vi "Calculate Output Sampling.vi"(10 "sampling info":cluster{"Fs":dbl, "#s":dbl}={"Fs"=204800.0, "#s"=20480.0}, 11 "Cfg_REF":T2 {"Roll-Off" min=1 max=4; "TC" min=1e-06 max=100.0 format="%#_3p"; "Phase" format="%#_3p"; "Frequency" min=1e-06 max=102400.0 format="%#_6p"; "Channel" min=1}) -> (2 "Filter Parameters":T1, 3 "Cfg_REF out":T2 {"Roll-Off" min=1 max=4; "TC" min=1e-06 max=100.0 format="%#_3p"; "Phase" format="%#_3p"; "Frequency" min=1e-06 max=102400.0 format="%#_6p"; "Channel" min=1})   [LabVIEW 2019, in "Instrument.Lockin.lvlib" / "Instrument.Lockin.lvclass"]
uses:
  Instrument.Lockin.lvclass
  Instrument.DAQ/Typedefs/REF.Channel--Cluster--Array.ctl
  Instrument.DAQ/Typedefs/REF.Channel--Cluster.ctl
  DSP/DSP.lvclass
  Instrument.DAQ/Instrument.DAQ.lvclass
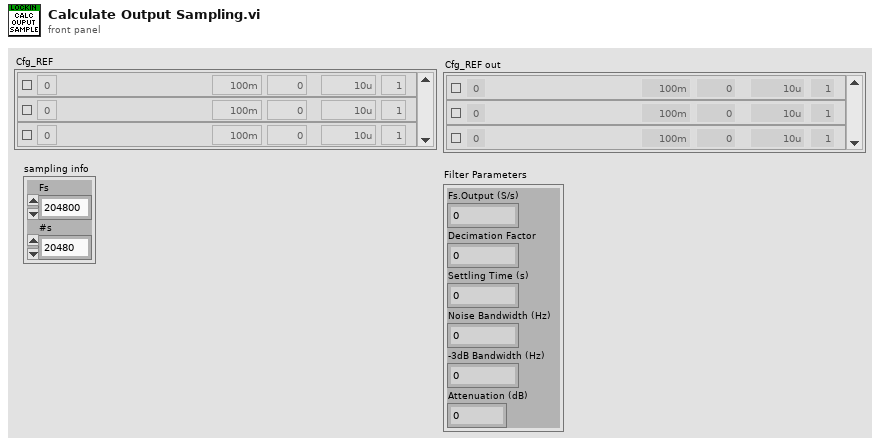
[diagram p1: front panel]
types:
  T1 = cluster{"Fs.Output (S/s)":dbl, "Decimation Factor":i32, "Settling Time (s)":dbl, "Noise Bandwidth (Hz)":dbl, "-3dB Bandwidth (Hz)":dbl, "Attenuation (dB)":dbl}
  T2 = typedef "Instrument.Lockin.lvlib/Instrument.DAQ.lvclass/REF.Channel--Cluster--Array.ctl" = T3[]
  T3 = typedef "Instrument.Lockin.lvlib/Instrument.DAQ.lvclass/REF.Channel--Cluster.ctl" = cluster{"Enable?":bool, "Channel":i32, "Frequency":dbl, "Phase":dbl, "TC":dbl, "Roll-Off":i32}
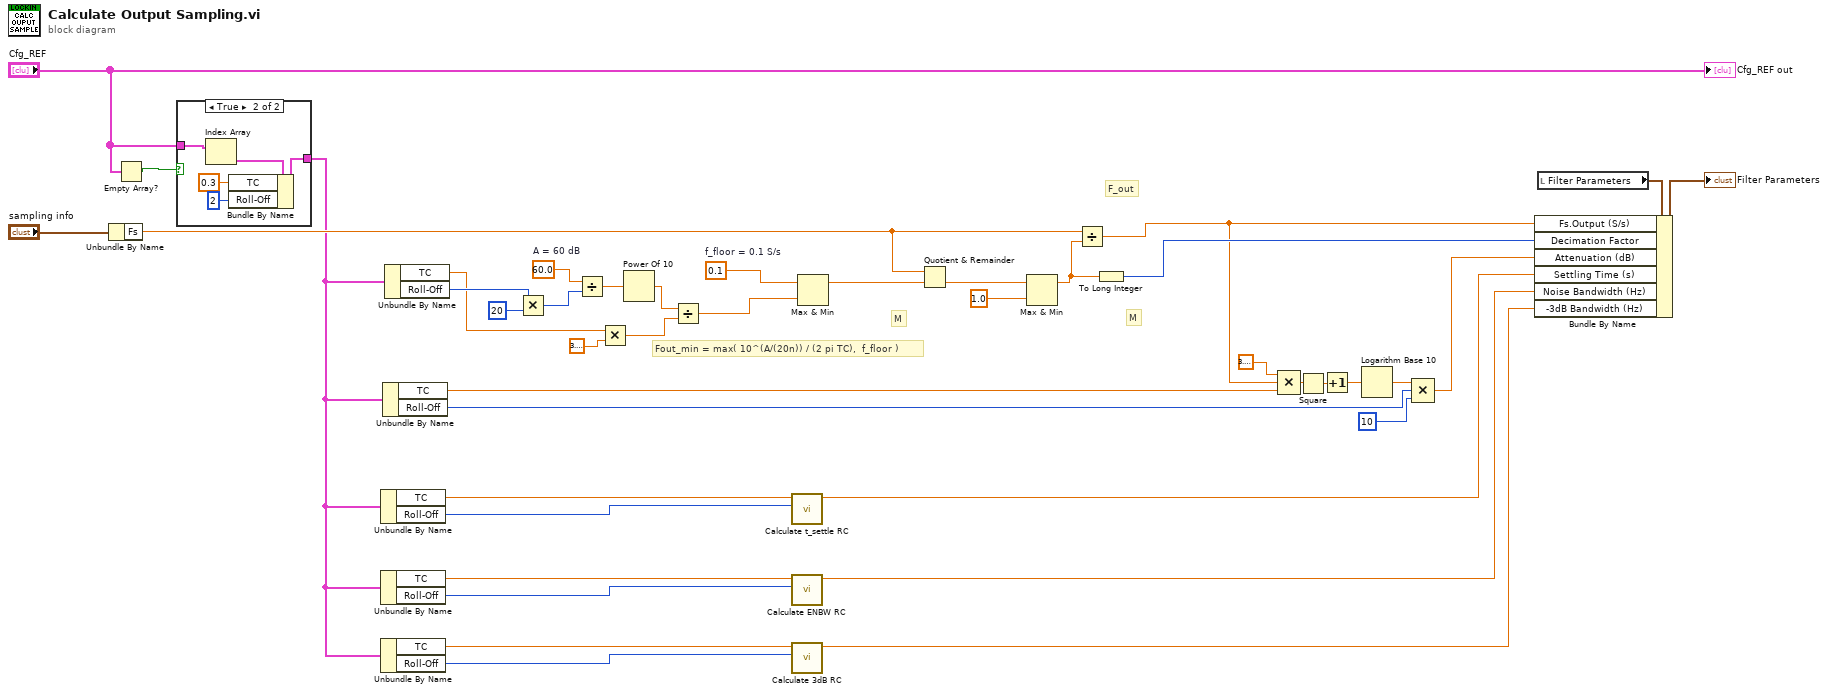
[diagram p0: block diagram]
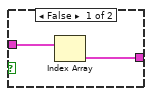
[diagram p2: hidden frame]
diagram:
  w20 = 60.0  # A = 60 dB
  w25 = 0.1  # f_floor = 0.1 S/s
  # "M"
  # "F_out"
  # "Fout_min = max( 10^(A/(20n)) / (2 pi TC),  f_floor )"
  # "M"
  n1 = Unbundle By Name("sampling info") -> ("Fs"=w36:dbl)
  n2 = Empty Array?(array="Cfg_REF") -> (empty?=w5:bool)
  n3 = case shown="True" w5 {
    tunnel: "Cfg_REF" -> [w44 w48]
    tunnel: [w43 w49] -> w32
    frame False {
      n4 = Index Array(array=w44) -> (element=w43:T3)  [unwired: 1 in]
    }
    frame True {
      n5 = Index Array(array=w48) -> (element=w47:T3)  [unwired: 1 in]
      n6 = Bundle By Name(cluster=w47, "TC"=0.3, "Roll-Off"=2) -> (w49:T3)
    }
  }
  n7 = Unbundle By Name(w32) -> ("TC"=w27:dbl, "Roll-Off"=w26:i32)
  n8 = Unbundle By Name(w32) -> ("TC"=w29:dbl, "Roll-Off"=w28:i32)
  n9 = Unbundle By Name(w32) -> ("TC"=w31:dbl, "Roll-Off"=w30:i32)
  n10 = Unbundle By Name(w32) -> ("TC"=w13:dbl, "Roll-Off"=w8:i32)
  n11 = Unbundle By Name(w32) -> ("TC"=w19:dbl, "Roll-Off"=w24:i32)
  n12 = Multiply(x=w24, y=20) -> (x*y=w21:i32)
  n13 = Divide(x=w20, y=w21) -> (x/y=w22:dbl)
  n14 = Multiply(x=w19, y=3.141592653589793) -> (x*y=w16:dbl)
  n15 = Power Of 10(x=w22) -> (10^x=w17:dbl)
  n16 = Divide(x=w17, y=w16) -> (x/y=w15:dbl)
  n17 = call "Calculate t_settle RC.vi"("filter order"=w26, "time constant (s)"=w27) -> ("f -3 dB (Hz)"=w38:dbl)  [unwired: 9 in]
  n18 = call "Calculate ENBW RC.vi"("filter order"=w28, "time constant (s)"=w29) -> ("ENBW (Hz)"=w39:dbl)  [unwired: 9 in]
  n19 = call "Calculate 3dB RC.vi"("filter order"=w30, "time constant (s)"=w31) -> ("f -3 dB (Hz)"=w40:dbl)  [unwired: 9 in]
  n20 = Max & Min(x=w25, y=w15) -> (max(x,y)=w14:dbl)  [unwired: 1 out]
  n21 = Quotient & Remainder(x=w36, y=w14) -> (floor(x/y)=w3:dbl)  [unwired: 1 out]
  n22 = Max & Min(x=w3, y=1.0 ("lower limit")) -> (max(x,y)=w2:dbl)  [unwired: 1 out]
  n23 = Divide(x=w36, y=w2) -> (x/y=w33:dbl)
  n24 = To Long Integer(number=w2) -> (32bit integer=w34:i32)
  n25 = Compound Arithmetic op=MULTIPLY(3.141592653589793, w33, w13) -> (w11:dbl)
  n26 = Square(x=w11) -> (x^2=w6:dbl)
  n27 = Increment(x=w6) -> (x+1=w10:dbl)
  n28 = Logarithm Base 10(1:w10) -> (0:w9:dbl)
  n29 = Compound Arithmetic op=MULTIPLY(w9, w8, 10 ("y")) -> (w37:dbl)
  n30 = local read "Filter Parameters"() -> (w42:T1)
  n31 = Bundle By Name(cluster=w42, "Fs.Output (S/s)"=w33, "Decimation Factor"=w34, "Attenuation (dB)"=w37, "Settling Time (s)"=w38, "Noise Bandwidth (Hz)"=w39, "-3dB Bandwidth (Hz)"=w40) -> (→"Filter Parameters":T1)
  "Cfg_REF out" <- "Cfg_REF"
